vi "Add Receiver Group.vi"(8 "error in (no error)":errorcluster caption="错误输入（无错误）", 10 "Receiver Group":string[](array[string]), 11 "Email In":refnum<class "Email.lvclass"> caption="DNL_LabVIEW Object in") -> (0 "error out":errorcluster caption="错误输出", 3 "Email Out":refnum<class "Email.lvclass"> caption="DNL_LabVIEW Object out")   [LabVIEW 2012, in "Email.lvclass"]
uses:
  Email.lvclass
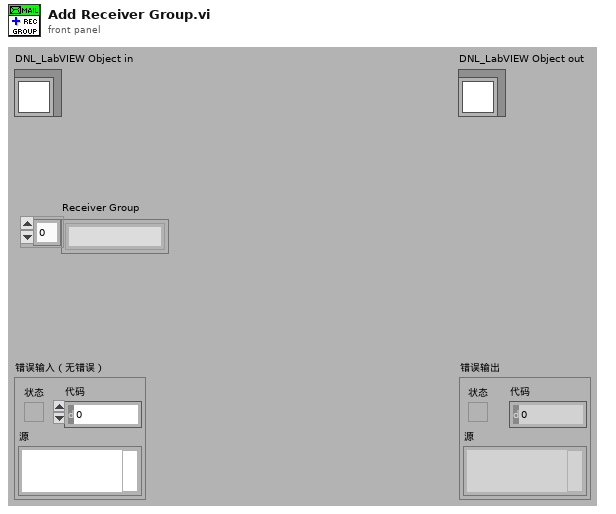
[diagram p1: front panel]
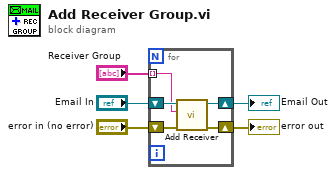
[diagram p0: block diagram]
diagram:
  n1 = for {
    shift-right: [w9] -> w4
    shift-left: "Email In" -> [w10]
    shift-right: [w7] -> w2
    shift-left: "error in (no error)" -> [w8]
    tunnel: "Receiver Group" -> [w6] mode=indexing
    n2 = call "Add Receiver.vi"("error in (no error)"=w8, "Receiver Address"=w6, "Email In"=w10) -> ("error out"=w7:errorcluster, "Email Out"=w9:refnum<class "Email.lvclass">)  [unwired: 7 in]
  }
  "error out" <- w2
  "Email Out" <- w4
